vi "PH_HamamatsuCamera.set modified data.vi"(0 "i ref in":refnum<vi>, 2 "i attribute":T1={"Gui Refs"={"Camera Details"=refnum, "ROI"=refnum, "Set ROI to Maximum"=refnum, "Trigger Parameters"=refnum, "Brightness"=refnum, "Shutter"=refnum, "Gain"=refnum, "Trigger Timeout"=refnum, "Trigger Polarity"=refnum, "Trigger Mode"=refnum, "Parameters"=refnum, "Set Cam Parameter"=refnum, "Parameter to set"=refnum, "Value to set"=refnum}, "Cam"={"Handle"=-1, "Details"={"Model"="", "Camera ID"="", "Firmware"=""}, "Buffer Info"={"height"=0, "width"=0, "datatype"=0}}, "H Offset"={"Value"=0, "Minimum"=0, "Maximum"=0, "Increment"=0}, "V Offset"={"Value"=0, "Minimum"=0, "Maximum"=0, "Increment"=0}, "H Width"={"Value"=0, "Minimum"=0, "Maximum"=0, "Increment"=0}, "V Width"={"Value"=0, "Minimum"=0, "Maximum"=0, "Increment"=0}, "Trigger Parameters"={"Mode"=1, "Polarity"=1, "Times"=1, "Delay"=0.0}, "Trigger Timeout"=1000, "Parameters"=[], "Indicees Cam Parameters"={"Brightness"=-1, "Shutter"=-1, "Gain"=-1}, "Wanted Values"={"Trigger Settings"=[], "ROI"=[], "Parameter"=[]}} {"Wanted Values"."Trigger Settings"."Polarity" items=["Negative"=1, "Positive"=2]; "Wanted Values"."Trigger Settings"."Mode" items=["Internal"=1, "External Edge"=2, "External Level"=4, "Software"=32, "Fast Repetition"=64, "TDI"=128, "Trigger Start"=512, "Sync Readout"=1024]; "Trigger Parameters"."Polarity" items=["Negative"=1, "Positive"=2]; "Trigger Parameters"."Mode" items=["Internal"=1, "External Edge"=2, "External Level"=4, "Software"=32, "Fast Repetition"=64, "TDI"=128, "Trigger Start"=512, "Sync Readout"=1024]}, 5 "error in (no error)":errorcluster) -> (14 "i ref out":refnum<vi>, 19 "error out":errorcluster)   [LabVIEW 2014, in "PH_HamamatsuCamera.lvlib"]
doc: "Writes the data into the attribute of an object. Then, the attribute dara are unlocked using the \"release\" method. Prior to calling THIS method, the attribute data must have been locked using the methods \"lock\" or \"get data to modify\".\n\n\nLicense Agreement for this software:\n\nCopyright (C)\nGesellschaft für Schwerionenforschung, GSI\nPlanckstr. 1\n64291 Darmstadt\nGermany\n\nContact: D.Beck@gsi.de \n\nThis program is free software; you can redistribute it and/or modify it under the terms of the GNU General Public License as published by the Free Software Foundation; either version 2 of the license, or (at your option) any later version.\n\nThis program is distributed in the hope that it will be useful, but WITHOUT ANY WARRANTY; without even the implied warranty of MERCHANTABILITY or FITNESS FOR A PARTICULAR PURPOSE. See the GNU General License for more details (http://www.gnu.org).\n\nGesellschaft für Schwerionenforschung, GSI\nPlanckstr. 1, 64291 Darmstadt, Germany\nFor all questions and ideas contact: M.Richter@gsi.de, H.Brand@gsi.de or D.Beck@gsi.de.\nLast update: 17-JUN-2004"
uses:
  PH_HamamatsuCamera.lvlib
  PH_HamamatsuCamera.i attribute.ctl
  PH_HamamatsuCamera.Trigger Parameter.ctl
  PH_HamamatsuCamera.Parameter Set.ctl
  PH_HamamatsuCamera.ROI.ctl
  CSCore/CSObj/CSObj.lvlib
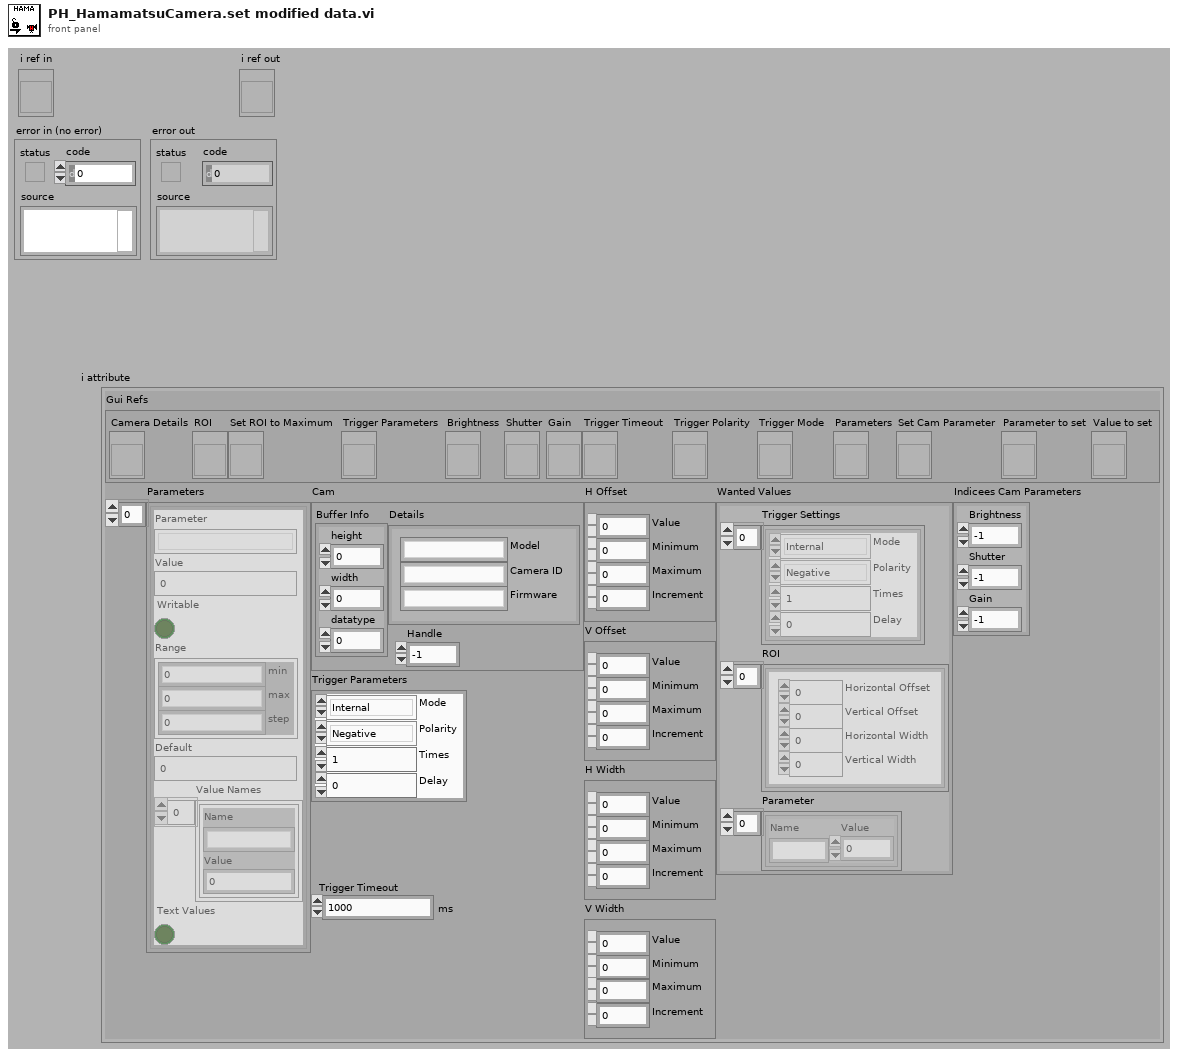
[diagram p1: front panel]
types:
  T1 = typedef "PH_HamamatsuCamera.lvlib/PH_HamamatsuCamera.i attribute.ctl" = cluster{"Gui Refs":cluster{"Camera Details":refnum<vi>, "ROI":refnum<vi>, "Set ROI to Maximum":refnum<vi>, "Trigger Parameters":refnum<vi>, "Brightness":refnum<vi>, "Shutter":refnum<vi>, "Gain":refnum<vi>, "Trigger Timeout":refnum<vi>, "Trigger Polarity":refnum<vi>, "Trigger Mode":refnum<vi>, "Parameters":refnum<vi>, "Set Cam Parameter":refnum<vi>, "Parameter to set":refnum<vi>, "Value to set":refnum<vi>}, "Cam":cluster{"Handle":i32, "Details":cluster{"Model":string, "Camera ID":string, "Firmware":string}, "Buffer Info":cluster{"height":u32, "width":u32, "datatype":u32}}, "H Offset":cluster{"Value":i32, "Minimum":i32, "Maximum":i32, "Increment":i32}, "V Offset":cluster{"Value":i32, "Minimum":i32, "Maximum":i32, "Increment":i32}, "H Width":cluster{"Value":i32, "Minimum":i32, "Maximum":i32, "Increment":i32}, "V Width":cluster{"Value":i32, "Minimum":i32, "Maximum":i32, "Increment":i32}, "Trigger Parameters":T2, "Trigger Timeout":u32, "Parameters":T3[], "Indicees Cam Parameters":cluster{"Brightness":i32, "Shutter":i32, "Gain":i32}, "Wanted Values":cluster{"Trigger Settings":T2[], "ROI":T4[], "Parameter":cluster{"Name":string, "Value":dbl}[]}}
  T2 = typedef "PH_HamamatsuCamera.lvlib/PH_HamamatsuCamera.Trigger Parameter.ctl" = cluster{"Mode":u32, "Polarity":u32, "Times":u32, "Delay":dbl}
  T3 = typedef "PH_HamamatsuCamera.lvlib/PH_HamamatsuCamera.Parameter Set.ctl" = cluster{"Parameter":string, "Value":dbl, "Writable":bool, "Range":cluster{"min":dbl, "max":dbl, "step":dbl}, "Default":dbl, "Value Names":cluster{"Name":string, "Value":dbl}[], "Text Values":bool}
  T4 = typedef "PH_HamamatsuCamera.lvlib/PH_HamamatsuCamera.ROI.ctl" = cluster{"Horizontal Offset":i32, "Vertical Offset":i32, "Horizontal Width":i32, "Vertical Width":i32}
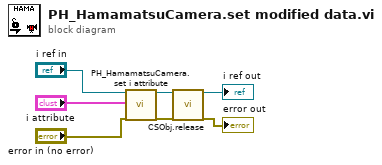
[diagram p0: block diagram]
diagram:
  n1 = call "PH_HamamatsuCamera.set i attribute.vi"("i ref in"="i ref in", "i attribute"="i attribute", "error in (no error)"="error in (no error)") -> ("i ref out"=w4:refnum<vi>, "error out"=w3:errorcluster)  [unwired: 15 in]
  n2 = call "CSObj.release.vi"("i ref in"=w4, "error in (no error)"=w3) -> ("i ref out"=→"i ref out":refnum<vi>, "error out"=→"error out":errorcluster)  [unwired: 16 in]
